vi "UserAccessLog.vi"(11 "Active User":string) -> ()   [LabVIEW 2023]
uses:
  TypeDefs/Paths/UsersLogPath.ctl
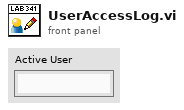
[diagram p1: front panel]
types:
  T1 = enum16{"open", "replace", "create", "open or create", "replace or create", "replace or create with confirmation"}
  T2 = typedef "UsersLogPath.ctl" = path
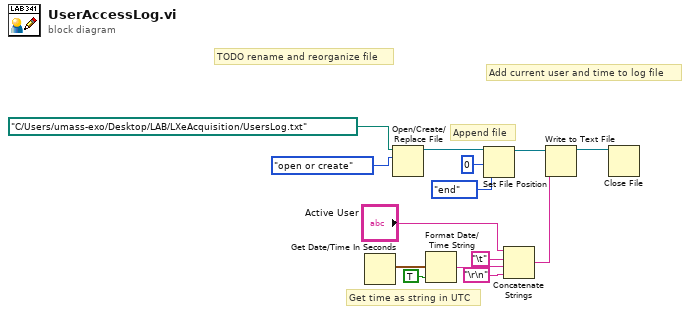
[diagram p0: block diagram]
diagram:
  # "Append file"
  # "Add current user and time to log file"
  # "TODO rename and reorganize file"
  # "Get time as string in UTC"
  n1 = Get Date/Time In Seconds() -> (seconds since 1Jan1904=w13:timestamp)
  n2 = Open/Create/Replace File(file path (use dialog)=T2 path "C:/Users/umass-exo/Desktop/LAB/LXeAcquisition/UsersLog.txt", operation (0:open)=T1."open or create") -> (refnum out=w4:refnum<file>)  [unwired: 4 in, 2 out]
  n3 = Format Date/Time String(seconds (now)=w13, UTC format=TRUE) -> (date/time string=w11:string)  [unwired: 1 in]
  n4 = Set File Position(offset (in bytes) (0)=i64 0, refnum=w4, from (0:start)=enum16{"start", "end", "current"}."end") -> (refnum out=w3:refnum<file>)  [unwired: 1 in, 1 out]
  n5 = Concatenate Strings("Active User", "\t", w11, "\r\n") -> (w9:string)
  n6 = Write to Text File(file (use dialog)=w3, text=w9) -> (refnum out=w14:refnum<file>)  [unwired: 2 in, 2 out]
  n7 = Close File(refnum=w14) -> ()  [unwired: 1 in, 2 out]
